vi "Stop Bit.vi"(8 "error in (no error)":errorcluster, 11 "Low Speed in":refnum<class "Low Speed.lvclass">) -> (0 "error out":errorcluster, 3 "Low Speed out":refnum<class "Low Speed.lvclass">)   [LabVIEW 2020, in "Low Speed.lvclass"]
uses:
  Low Speed.lvclass
  C:/Users/kaiser.asan/OneDrive - SolitonTechnologies/LabVIEW/29.SDLC - I2C Driver/I2C Module/I2C Controller Module/Class/Transmission Mode/Parent/TX Speed.lvclass
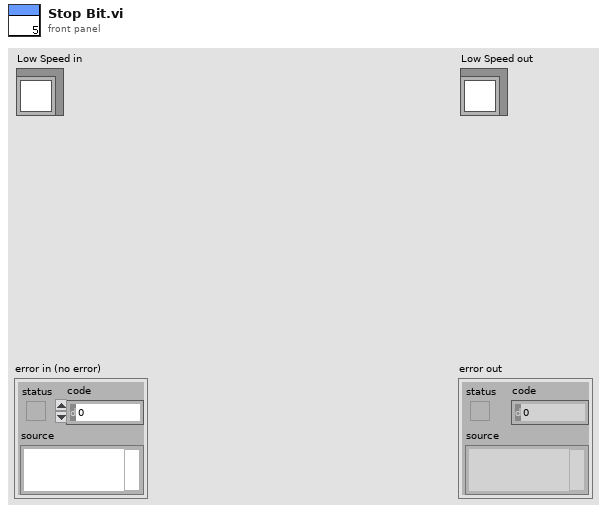
[diagram p1: front panel]
types:
  T1 = typedef "I2C Controller Lib.lvlib/Timing Parameters Cluster.ctl" = cluster{"f_SCL(KHz)":u32, "t_HIGH (ns)":u32, "t_LOW (ns)":u32, "t_SU;STA (ns)":u32, "t_HD;STA (ns)":u32, "t_SU;DAT (ns)":u32, "t_HD;DAT (ns)":u32, "t_SU;STO (ns)":u32, "t_BUF (ns)":u32}
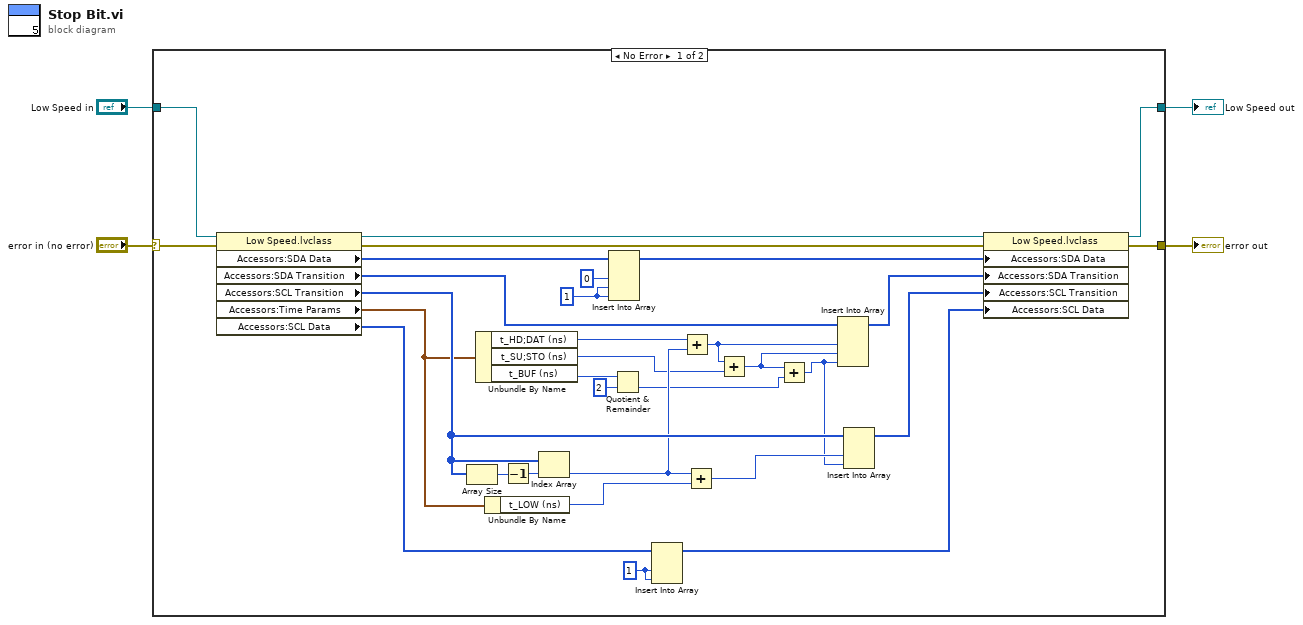
[diagram p0: block diagram]
diagram:
  n1 = case shown="No Error" "error in (no error)" {
    selector: "error in (no error)" -> [w35 w37]
    tunnel: [w32 w37] -> w4
    tunnel: [w30 w36] -> w2
    tunnel: "Low Speed in" -> [w33 w36]
    frame No Error {
      w13 = u8 1 ("new element/subarray")
      w7 = u8 1 ("new element/subarray")
      n2 = property class="Low Speed.lvclass"(reference=w33, error in=w35) -> (reference out=w31:refnum<class "Low Speed.lvclass">, error out=w34:errorcluster, "Accessors:SDA Data"=w29:u8[], "Accessors:SDA Transition"=w27:u32[], "Accessors:SCL Transition"=w21:u32[], "Accessors:Time Params"=w20:T1, "Accessors:SCL Data"=w5:u8[])
      n3 = Array Size(array=w21) -> (size(s)=w24:i32)
      n4 = Unbundle By Name(w20) -> ("t_HD;DAT (ns)"=w25:u32, "t_SU;STO (ns)"=w12:u32, "t_BUF (ns)"=w16:u32)
      n5 = Unbundle By Name(w20) -> ("t_LOW (ns)"=w22:u32)
      n6 = Decrement(x=w24) -> (x-1=w23:i32)
      n7 = Index Array(array=w21, index=w23) -> (element=w14:u32)
      n8 = Insert Into Array(array=w29, new element #1=u8 0 ("new element/subarray"), new element #2=w13, new element #3=w13) -> (w28:u8[])  [unwired: 1 in]
      n9 = Quotient & Remainder(x=w16, y=u32 2) -> (floor(x/y)=w9:u32)  [unwired: 1 out]
      n10 = Insert Into Array(array=w5, new element #1=w7, new element #2=w7) -> (w18:u8[])  [unwired: 1 in]
      n11 = Add(x=w25, y=w14) -> (x+y=w8:u32)
      n12 = Add(x=w14, y=w22) -> (x+y=w11:u32)
      n13 = Add(x=w8, y=w12) -> (x+y=w10:u32)
      n14 = Add(x=w10, y=w9) -> (x+y=w6:u32)
      n15 = Insert Into Array(array=w27, new element #1=w8, new element #2=w10, new element #3=w6) -> (w26:u32[])  [unwired: 1 in]
      n16 = Insert Into Array(array=w21, new element #1=w11, new element #2=w6) -> (w19:u32[])  [unwired: 1 in]
      n17 = property class="Low Speed.lvclass"(reference=w31, error in=w34, "Accessors:SDA Data"=w28, "Accessors:SDA Transition"=w26, "Accessors:SCL Transition"=w19, "Accessors:SCL Data"=w18) -> (reference out=w30:refnum<class "Low Speed.lvclass">, error out=w32:errorcluster)
    }
    frame Error {
    }
  }
  "error out" <- w4
  "Low Speed out" <- w2
